vi "Open 2601B.vi"() -> (0 "错误输出":errorcluster, 3 "VISA资源名称输出":refnum<visa-resource-name>)   [LabVIEW 2020]
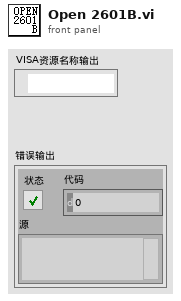
[diagram p1: front panel]
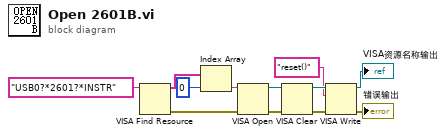
[diagram p0: block diagram]
diagram:
  n1 = VISA Find Resource(11:"USB0?*2601?*INSTR" ("表达式(\"?*\")")) -> (0:w5:errorcluster, 3:w3:string[])  [unwired: 2 in, 1 out]
  n2 = Index Array(array=w3, index=0 ("索引")) -> (element=w1:string)
  n3 = VISA Open(error in (no error)=w5, VISA resource name=w1) -> (VISA resource name=w12:refnum<visa-resource-name>, error out=w11:errorcluster)  [unwired: 3 in]
  n4 = VISA Clear(VISA resource name=w12, error in (no error)=w11) -> (VISA resource name out=w10:refnum<visa-resource-name>, error out=w9:errorcluster)
  n5 = VISA Write(VISA resource name=w10, write buffer="reset()" ("写入缓冲区"), error in (no error)=w9) -> (VISA resource name out=→"VISA资源名称输出":refnum<visa-resource-name>, error out=→"错误输出":errorcluster)  [unwired: 1 out]
